vi "TCP-Find Next Available Port.vi"(0 "net address":u32, 5 "start":u16=4900) -> (6 "port":u16, 15 "error out":errorcluster)   [LabVIEW 2020]
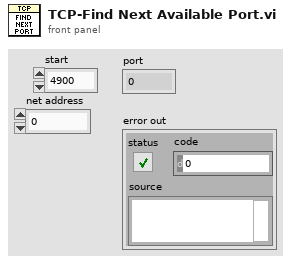
[diagram p1: front panel]
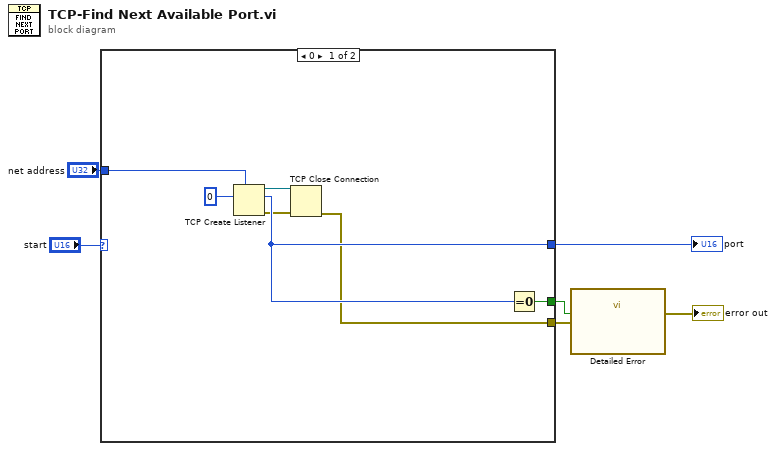
[diagram p0: block diagram]
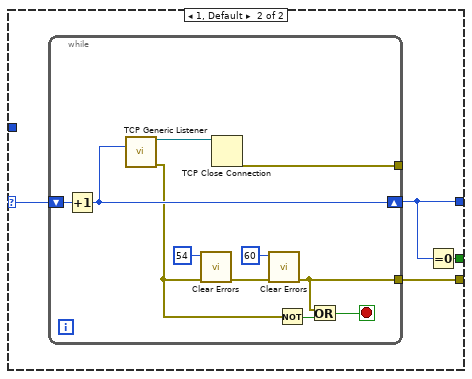
[diagram p2: hidden frame]
diagram:
  n1 = case shown="0" "start" {
    selector: "start" -> [_ w17]
    tunnel: [w10 w16] -> w5
    tunnel: [w7 w15] -> w4
    tunnel: [w11 w14] -> w3
    tunnel: "net address" -> [w13 _]
    frame 0 {
      n2 = TCP Create Listener(7:w13, 10:u16 0 ("port")) -> (0:w8:errorcluster, 2:w10:u16, 3:w9:refnum<k5>)  [unwired: 3 in]
      n3 = TCP Close Connection(connection ID=w9, error in (no error)=w8) -> (error out=w7:errorcluster)  [unwired: 1 in, 1 out]
      n4 = Equal To 0?(x=w10) -> (x = 0?=w11:bool)
    }
    frame 1, Default {
      n5 = while {
        tunnel: [w19] -> w15
        tunnel: [w27] -> _
        shift-right: [w23] -> w16
        shift-left: w17 -> [w28]
        stop <- w24 stop-if-true
        n6 = Increment(x=w28) -> (x+1=w23:u16)
        n7 = call "TCP Generic Listener.vi"("port"=w23) -> ("connection ID"=w22:refnum<k5>, "error out"=w21:errorcluster)  [unwired: 12 in, 1 out]
        n8 = call <vilib>:"Clear Errors.vi"("error in (no error)"=w21, "specific error code to clear (0: all)"=54) -> ("error out"=w20:errorcluster)  [unwired: 4 in, 1 out]
        n9 = TCP Close Connection(connection ID=w22) -> (error out=w27:errorcluster)  [unwired: 2 in, 1 out]
        n10 = call <vilib>:"Clear Errors.vi"("error in (no error)"=w20, "specific error code to clear (0: all)"=60) -> ("error out"=w19:errorcluster)  [unwired: 4 in, 1 out]
        n11 = Not(x=w21) -> (.not. x?=w25:bool)
        n12 = Or(x=w19, y=w25) -> (x .or. y?=w24:bool)
      }
      n13 = Equal To 0?(x=w16) -> (x = 0?=w14:bool)
    }
  }
  "port" <- w5
  n14 = call "Detailed Error"("Error?"=w3, "Primary"=w4) -> ("detailed error"=→"error out":errorcluster)  [unwired: 13 in]
